vi "rqcBob Photon Detector (FPGA).vi"(0 "detector signal in":bool, 1 "current cycle":u8, 2 "reset":bool, 9 "detector.detector window":u16, 12 "detector.use detector window":bool) -> (4 "detector out":bool)   [LabVIEW 2018]
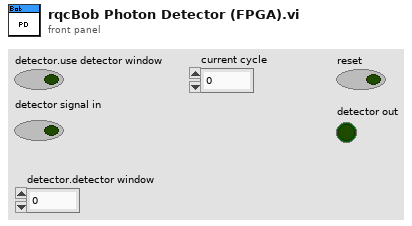
[diagram p1: front panel]
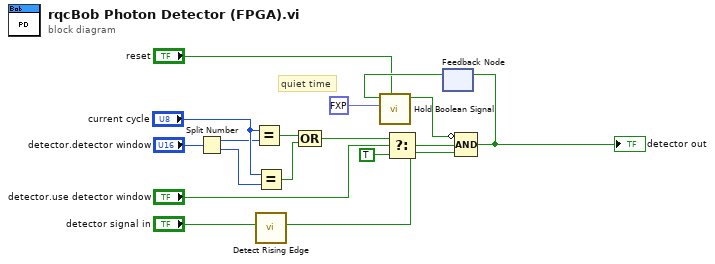
[diagram p0: block diagram]
diagram:
  # "quiet time"
  n1 = Split Number(x="detector.detector window") -> (hi(x)=w6:u8, lo(x)=w5:u8)
  n2 = Equal?(x="current cycle", y=w6) -> (x = y?=w12:bool)
  n3 = Equal?(x="current cycle", y=w5) -> (x = y?=w11:bool)
  n4 = call <vilib>:"Detect Rising Edge.vi"("signal"="detector signal in") -> ("edge detected"=w16:bool)  [unwired: 10 in]
  n5 = Compound Arithmetic op=OR(w12, w11) -> (w10:bool)
  n6 = Select(t=w10, s="detector.use detector window", f=TRUE ("value")) -> (s? t:f=w14:bool)
  n7 = feedback #1() -> (w8:bool)  [unwired: 1 in]
  n8 = call <vilib>:"Hold Boolean Signal.vi"("reset"="reset", "width"=fxp<+,5,5> 31.0, "input signal"=w8) -> ("output signal"=w3:bool)  [unwired: 8 in]
  n9 = Compound Arithmetic op=AND(invert w3, w14, w16) -> (w1:bool)
  "detector out" <- w1
  n10 = feedback-in #1(w1) -> ()
